vi "SCCSup Listbox_GetSymbol.vi"(0 "operation":T1(ring), 2 "symbol in":i32) -> (6 "symbol out":i32)   [LabVIEW 2017]
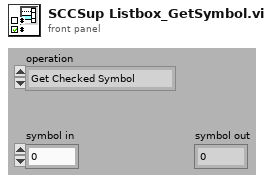
[diagram p1: front panel]
types:
  T1 = enum16{"Get Checked Symbol", "Get Unchecked Symbol", "Toggle Symbol"}
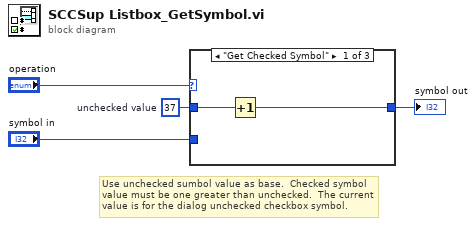
[diagram p0: block diagram]
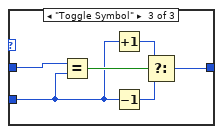
[diagram p3: hidden frame]
diagram:
  w1 = 37  # unchecked value
  # "Use unchecked sumbol value as base.  Checked symbol value must be one greater than unchecked.  The current value is for the dialog unchecked checkbox symbol."
  n1 = case shown="\"Get Checked Symbol\"" "operation" {
    tunnel: w1 -> [w6 w7 w13]
    tunnel: [w5 w7 w11] -> w3
    tunnel: "symbol in" -> [_ _ w10]
    frame "Get Checked Symbol" {
      n2 = Increment(x=w6) -> (x+1=w5:i32)
    }
    frame "Get Unchecked Symbol", Default {
    }
    frame "Toggle Symbol" {
      n3 = Equal?(x=w13, y=w10) -> (x = y?=w12:bool)
      n4 = Increment(x=w10) -> (x+1=w8:i32)
      n5 = Decrement(x=w10) -> (x-1=w9:i32)
      n6 = Select(t=w8, s=w12, f=w9) -> (s? t:f=w11:i32)
    }
  }
  "symbol out" <- w3
